vi "Autonomous Independent.vi"() -> ()   [LabVIEW 2017]
doc: "This VI is called when autonomous begins, and will automatically be terminated when autonomous ends. You can carry out timed or sensor driven robot movement independently without needing to return to the caller."
uses:
  <vilib>/Rock Robotics/WPI/ThirdParty/Phoenix-LabVIEW/Motor Controller/Controls/CTRE_Phoenix_MotorControl_ControlMode.ctl
  <vilib>/Rock Robotics/WPI/Utilities/WPI_GetSetVariantRefNum.vi
  <vilib>/Rock Robotics/Network Tables/NT Read String.vi
  <vilib>/Rock Robotics/Network Tables/NT Write Numeric Array.vi
panel:
  in  "Output 6":dbl
  in  "Output 4":dbl
  in  "Output 5":dbl
  in  "Output 3":dbl
  in  "Output 2":dbl
  in  "Ratio":dbl
  in  "Output":dbl
  in  "Ratio 2":dbl
  in  "Acceleration":i32=5000
  in  "Right CV":i32=2000
  in  "PIDF Motion Magic":cluster{"P":dbl, "I":dbl, "D":dbl, "F":dbl}={"P"=0.4, "I"=0.0, "D"=0.0, "F"=0.01}
  in  "Left CV":i32=4000
  # "Be sure to right-click and choose Data Operations>>Make Current Value default if you want to save the array values with the VI"
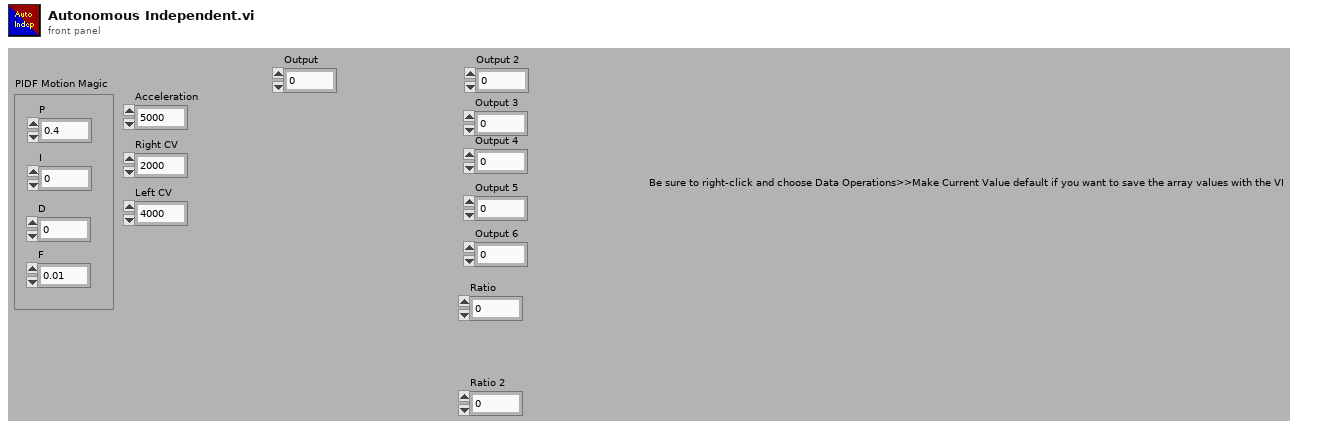
[diagram p1: front panel]
types:
  T1 = typedef "WPI_JoystickDevRef.ctl" = cluster{"Device":T2}
  T2 = typedef "WPI_JoystickDeviceEnum.ctl" = enum16{"USB 0", "USB 1", "USB 2", "USB 3", "USB 4", "USB 5"}
  T3 = typedef "WPI_MotorControlDeviceRef.ctl" = cluster{"DeviceStatus":errorcluster, "Type":T4, "PWM":cluster{"PWM Channel":T5, "DeadBand":T6}, "CAN":cluster{"Device Number":u8, "SetOutput VI Ref":variant, "GetOutput VI Ref":variant, "Enable VI Ref":variant, "Disable VI Ref":variant, "Data":variant}, "Invert":bool, "DIO PWM":cluster{"PWM \"Enable\" Channel":T5, "DIOChannel":T7, "PWM Rate":dbl}}
  T4 = typedef "WPI_MotorControlType.ctl" = enum16{"PWM", "CAN", "DIO PWM"}
  T5 = typedef "FPGA_DIOPWMChannel.ctl" = enum8{"PWM 0", "PWM 1", "PWM 2", "PWM 3", "PWM 4", "PWM 5", "PWM 6", "PWM 7", "PWM 8", "PWM 9", "PWM MXP 0", "PWM MXP 1", "PWM MXP 2", "PWM MXP 3", "PWM MXP 4", "PWM MXP 5", "PWM MXP 6", "PWM MXP 7", "PWM MXP 8", "PWM MXP 9", "Invalid"}
  T6 = typedef "WPI_PWMDeadband.ctl" = cluster{"Name":string, "maxPositivePwm":i32, "minPositivePwm":i32, "centerPwm":i32, "maxNegativePwm":i32, "minNegativePwm":i32, "angularRange":u16}
  T7 = typedef "FPGA_DIOChannel.ctl" = enum8{"DIO 0", "DIO 1", "DIO 2", "DIO 3", "DIO 4", "DIO 5", "DIO 6", "DIO 7", "DIO 8", "DIO 9", "DIO MXP 0", "DIO MXP 1", "DIO MXP 2", "DIO MXP 3", "DIO MXP 4", "DIO MXP 5", "DIO MXP 6", "DIO MXP 7", "DIO MXP 8", "DIO MXP 9", "DIO MXP 10", "DIO MXP 11", "DIO MXP 12", "DIO MXP 13", "DIO MXP 14", "DIO MXP 15", "SPI Port CS1", "SPI Port CS2", "SPI Port CS3", "SPI Port MISO", "SPI Port MOSI", "Invalid"}
  T8 = typedef "CTRE_Phoenix_MotorControl_ControlMode.ctl" = u16
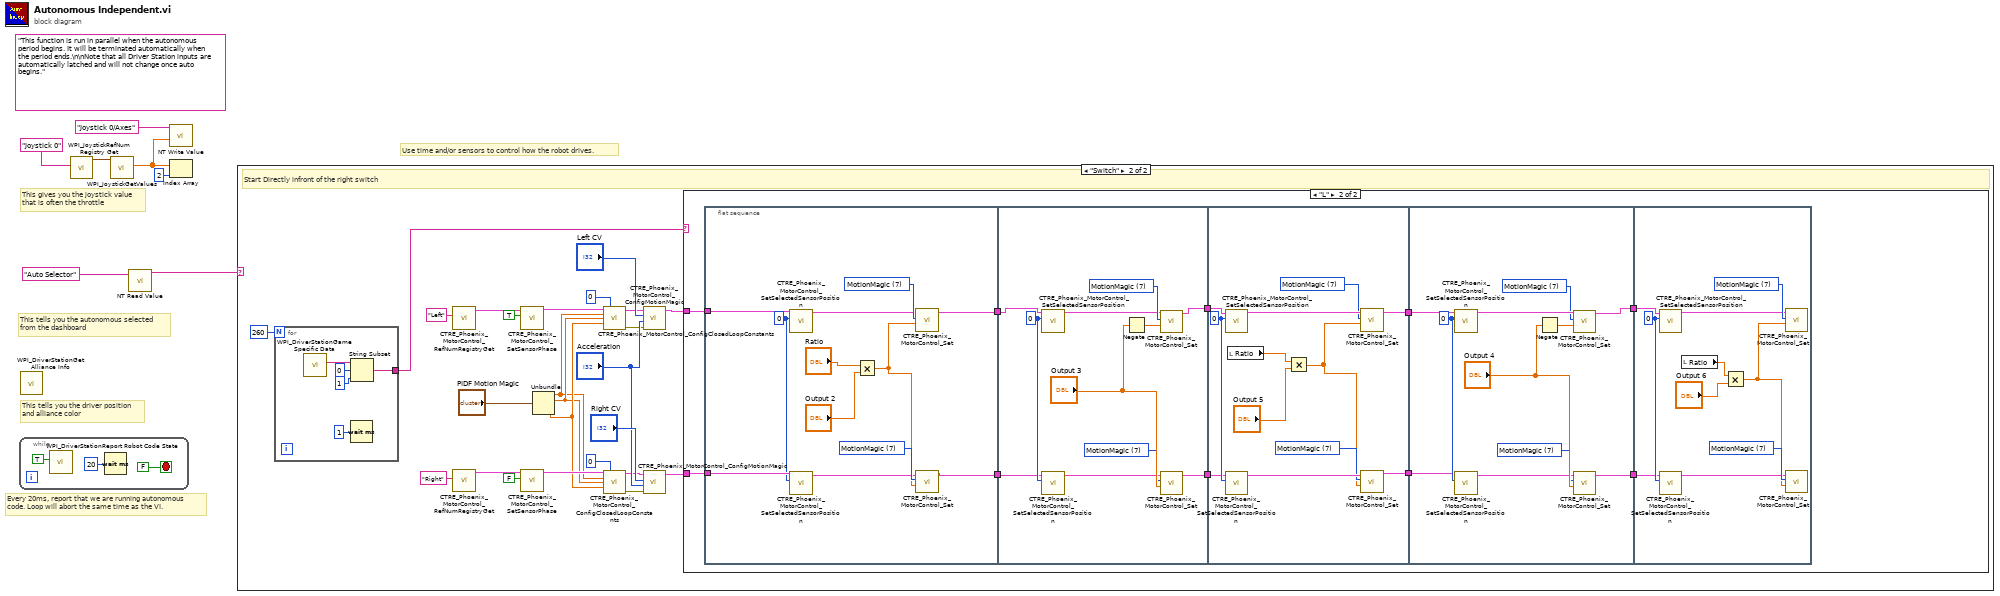
[diagram p0: block diagram]
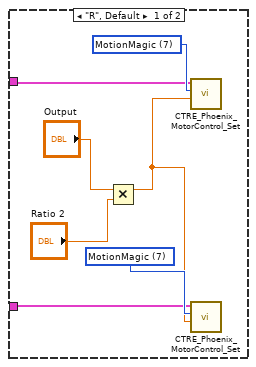
[diagram p3: hidden frame]
diagram:
  (unwired) "This function is run in parallel when the autonomous period begins. It will be terminated automatically when the period ends.\n\nNote that all Driver Station inputs are automatically latched and will not change once auto begins."
  # "This tells you the autonomous selected\nfrom the dashboard"
  # "Every 20ms, report that we are running autonomous\ncode. Loop will abort the same time as the VI."
  # "This gives you the joystick value\nthat is often the throttle"
  # "Use time and/or sensors to control how the robot drives."
  # "This tells you the driver position\nand alliance color"
  n1 = while {
    stop <- FALSE stop-if-true
    n2 = call <vilib>:"WPI_DriverStationReport Robot Code State.vi"("Autonomous"=TRUE) -> ()  [unwired: 10 in, 1 out]
    n3 = Wait (ms)(milliseconds to wait=u32 20) -> ()  [unwired: 1 out]
  }
  n4 = call <vilib>:"WPI_DriverStationGet Alliance Info.vi"() -> ()  [unwired: 12 out]
  n5 = call <vilib>:"WPI_JoystickRefNum Registry Get.vi"("refnum name"="Joystick 0") -> ("JoystickDevRef"=w6:T1)  [unwired: 1 in, 9 out]
  n6 = call <vilib>:"WPI_JoystickGetValues.vi"("JoystickDevRef"=w6) -> ("Axes"=w3:dbl[])  [unwired: 6 in, 4 out]
  n7 = call-poly <vilib>:"NT Read Value.vi"("Name"="Auto Selector") -> ("String"=w1:string)  [unwired: 9 in, 1 out]
  n8 = call-poly <vilib>:"NT Write Value.vi"("Numeric Array"=w3, "Name"="Joystick 0/Axes") -> ()  [unwired: 9 in, 1 out]
  n9 = Index Array(array=w3, index=2) -> ()  [unwired: 1 out]
  n10 = case shown="\"Switch\"" w1 {
    frame Default {
      # "You can put your main auto here, or you can right-click on the case and make any\nother frame be the default case."
      # "This is the frame that will execute if no selection is made, or if it is not recognized"
    }
    frame "Switch" {
      # "Start Directly infront of the right switch"
      n11 = for {
        N: 260 -> [_]
        tunnel: [w37] -> w35
        n12 = call <vilib>:"WPI_DriverStationGame Specific Data.vi"() -> ("Game Specific Data"=w40:string)  [unwired: 11 in]
        n13 = Wait (ms)(milliseconds to wait=u32 1) -> ()  [unwired: 1 out]
        n14 = String Subset(string=w40, offset (0)=0, length (rest)=1 ("length (rest)")) -> (substring=w37:string)
      }
      n15 = call "CTRE_Phoenix_MotorControl_RefNumRegistryGet.vi"("refnum name"="Left") -> ("PhoenixMotorControlDevRef"=w19:T3)  [unwired: 9 in, 1 out]
      n16 = call "CTRE_Phoenix_MotorControl_RefNumRegistryGet.vi"("refnum name"="Right") -> ("PhoenixMotorControlDevRef"=w20:T3)  [unwired: 9 in, 1 out]
      n17 = call "CTRE_Phoenix_MotorControl_SetSensorPhase.vi"("PhaseSensor"=TRUE, "PhoenixMotorControlDevRef"=w19) -> ("PhoenixMotorControlDevRef"=w33:T3)  [unwired: 8 in, 1 out]
      n18 = call "CTRE_Phoenix_MotorControl_SetSensorPhase.vi"("PhaseSensor"=FALSE, "PhoenixMotorControlDevRef"=w20) -> ("PhoenixMotorControlDevRef"=w32:T3)  [unwired: 8 in, 1 out]
      n19 = Unbundle("PIDF Motion Magic") -> ("P"=w25:dbl, "I"=w26:dbl, "D"=w27:dbl)  [unwired: 1 out]
      n20 = call "CTRE_Phoenix_MotorControl_ConfigClosedLoopConstants.vi"("PhoenixMotorControlDevRef"=w33, "slotIdx"=0, "P"=w25, "I"=w26, "D"=w27) -> ("PhoenixMotorControlDevRef"=w21:T3, "error out"=w22:errorcluster)  [unwired: 9 in]
      n21 = call "CTRE_Phoenix_MotorControl_ConfigClosedLoopConstants.vi"("PhoenixMotorControlDevRef"=w32, "slotIdx"=0, "P"=w25, "I"=w26, "D"=w27) -> ("PhoenixMotorControlDevRef"=w23:T3, "error out"=w24:errorcluster)  [unwired: 9 in]
      n22 = call "CTRE_Phoenix_MotorControl_ConfigMotionMagic.vi"("error in (no error)"=w22, "Acceleration"="Acceleration", "Cruise Velocity"="Left CV", "PhoenixMotorControlDevRef"=w21) -> ("PhoenixMotorControlDevRef"=w11:T3)  [unwired: 6 in, 1 out]
      n23 = call "CTRE_Phoenix_MotorControl_ConfigMotionMagic.vi"("error in (no error)"=w24, "Acceleration"="Acceleration", "Cruise Velocity"="Right CV", "PhoenixMotorControlDevRef"=w23) -> ("PhoenixMotorControlDevRef"=w12:T3)  [unwired: 6 in, 1 out]
      n24 = case shown="\"L\"" w35 {
        tunnel: w12 -> [w44 w57]
        tunnel: w11 -> [w43 w56]
        frame "R", Default {
          w46 = T8 7 items=["PercentOutput"=0, "Position"=1, "Velocity"=2, "Current"=3, "Follower"=5, "MotionProfile"=6, "MotionMagic"=7, "MotionMagicArc"=8, "MotionProfileArc"=10, "Disabled"=15] ("Control Mode")
          w45 = T8 7 items=["PercentOutput"=0, "Position"=1, "Velocity"=2, "Current"=3, "Follower"=5, "MotionProfile"=6, "MotionMagic"=7, "MotionMagicArc"=8, "MotionProfileArc"=10, "Disabled"=15] ("Control Mode")
          n25 = Multiply(x="Output", y="Ratio 2") -> (x*y=w42:dbl)
          n26 = call "CTRE_Phoenix_MotorControl_Set.vi"("Output"=w42, "Control Mode"=w45, "PhoenixMotorControlDevRef"=w43) -> ()  [unwired: 7 in, 2 out]
          n27 = call "CTRE_Phoenix_MotorControl_Set.vi"("Output"=w42, "Control Mode"=w46, "PhoenixMotorControlDevRef"=w44) -> ()  [unwired: 7 in, 2 out]
        }
        frame "L" {
          n28 = flat-sequence {
            tunnel: w57 -> [w63]
            tunnel: w56 -> [w65]
            tunnel: [w67] -> w55
            tunnel: [w66] -> w54
            tunnel: w55 -> [w72]
            tunnel: w54 -> [w75]
            tunnel: [w71] -> w51
            tunnel: [w70] -> w50
            tunnel: [w87] -> w53
            tunnel: [w86] -> w52
            tunnel: w51 -> [w85]
            tunnel: w50 -> [w84]
            tunnel: w53 -> [w96]
            tunnel: w52 -> [w95]
            tunnel: [w94] -> w49
            tunnel: [w93] -> w48
            tunnel: w49 -> [w108]
            tunnel: w48 -> [w107]
            frame #0 {
              w61 = 0 ("New Sensor Position")
              w69 = T8 7 items=["PercentOutput"=0, "Position"=1, "Velocity"=2, "Current"=3, "Follower"=5, "MotionProfile"=6, "MotionMagic"=7, "MotionMagicArc"=8, "MotionProfileArc"=10, "Disabled"=15] ("Control Mode")
              w68 = T8 7 items=["PercentOutput"=0, "Position"=1, "Velocity"=2, "Current"=3, "Follower"=5, "MotionProfile"=6, "MotionMagic"=7, "MotionMagicArc"=8, "MotionProfileArc"=10, "Disabled"=15] ("Control Mode")
              n29 = call "CTRE_Phoenix_MotorControl_SetSelectedSensorPosition.vi"("New Sensor Position"=w61, "PhoenixMotorControlDevRef"=w65) -> ("PhoenixMotorControlDevRef"=w64:T3)  [unwired: 8 in, 1 out]
              n30 = call "CTRE_Phoenix_MotorControl_SetSelectedSensorPosition.vi"("New Sensor Position"=w61, "PhoenixMotorControlDevRef"=w63) -> ("PhoenixMotorControlDevRef"=w62:T3)  [unwired: 8 in, 1 out]
              n31 = Multiply(x="Ratio", y="Output 2") -> (x*y=w59:dbl)
              n32 = call "CTRE_Phoenix_MotorControl_Set.vi"("Output"=w59, "Control Mode"=w68, "PhoenixMotorControlDevRef"=w64) -> ("PhoenixMotorControlDevRef"=w66:T3)  [unwired: 7 in, 1 out]
              n33 = call "CTRE_Phoenix_MotorControl_Set.vi"("Output"=w59, "Control Mode"=w69, "PhoenixMotorControlDevRef"=w62) -> ("PhoenixMotorControlDevRef"=w67:T3)  [unwired: 7 in, 1 out]
            }
            frame #1 {
              w76 = 0 ("New Sensor Position")
              w79 = T8 7 items=["PercentOutput"=0, "Position"=1, "Velocity"=2, "Current"=3, "Follower"=5, "MotionProfile"=6, "MotionMagic"=7, "MotionMagicArc"=8, "MotionProfileArc"=10, "Disabled"=15] ("Control Mode")
              w78 = T8 7 items=["PercentOutput"=0, "Position"=1, "Velocity"=2, "Current"=3, "Follower"=5, "MotionProfile"=6, "MotionMagic"=7, "MotionMagicArc"=8, "MotionProfileArc"=10, "Disabled"=15] ("Control Mode")
              n34 = call "CTRE_Phoenix_MotorControl_SetSelectedSensorPosition.vi"("New Sensor Position"=w76, "PhoenixMotorControlDevRef"=w75) -> ("PhoenixMotorControlDevRef"=w74:T3)  [unwired: 8 in, 1 out]
              n35 = call "CTRE_Phoenix_MotorControl_SetSelectedSensorPosition.vi"("New Sensor Position"=w76, "PhoenixMotorControlDevRef"=w72) -> ("PhoenixMotorControlDevRef"=w73:T3)  [unwired: 8 in, 1 out]
              n36 = Negate(x="Output 3") -> (-x=w77:dbl)
              n37 = call "CTRE_Phoenix_MotorControl_Set.vi"("Output"=w77, "Control Mode"=w78, "PhoenixMotorControlDevRef"=w74) -> ("PhoenixMotorControlDevRef"=w70:T3)  [unwired: 7 in, 1 out]
              n38 = call "CTRE_Phoenix_MotorControl_Set.vi"("Output"="Output 3", "Control Mode"=w79, "PhoenixMotorControlDevRef"=w73) -> ("PhoenixMotorControlDevRef"=w71:T3)  [unwired: 7 in, 1 out]
            }
            frame #2 {
              w92 = 0 ("New Sensor Position")
              w88 = T8 7 items=["PercentOutput"=0, "Position"=1, "Velocity"=2, "Current"=3, "Follower"=5, "MotionProfile"=6, "MotionMagic"=7, "MotionMagicArc"=8, "MotionProfileArc"=10, "Disabled"=15] ("Control Mode")
              w89 = T8 7 items=["PercentOutput"=0, "Position"=1, "Velocity"=2, "Current"=3, "Follower"=5, "MotionProfile"=6, "MotionMagic"=7, "MotionMagicArc"=8, "MotionProfileArc"=10, "Disabled"=15] ("Control Mode")
              n39 = call "CTRE_Phoenix_MotorControl_SetSelectedSensorPosition.vi"("New Sensor Position"=w92, "PhoenixMotorControlDevRef"=w84) -> ("PhoenixMotorControlDevRef"=w90:T3)  [unwired: 8 in, 1 out]
              n40 = call "CTRE_Phoenix_MotorControl_SetSelectedSensorPosition.vi"("New Sensor Position"=w92, "PhoenixMotorControlDevRef"=w85) -> ("PhoenixMotorControlDevRef"=w91:T3)  [unwired: 8 in, 1 out]
              n41 = local read "Ratio"() -> (w81:dbl)
              n42 = Multiply(x=w81, y="Output 5") -> (x*y=w82:dbl)
              n43 = call "CTRE_Phoenix_MotorControl_Set.vi"("Output"=w82, "Control Mode"=w89, "PhoenixMotorControlDevRef"=w90) -> ("PhoenixMotorControlDevRef"=w87:T3)  [unwired: 7 in, 1 out]
              n44 = call "CTRE_Phoenix_MotorControl_Set.vi"("Output"=w82, "Control Mode"=w88, "PhoenixMotorControlDevRef"=w91) -> ("PhoenixMotorControlDevRef"=w86:T3)  [unwired: 7 in, 1 out]
            }
            frame #3 {
              w99 = 0 ("New Sensor Position")
              w98 = T8 7 items=["PercentOutput"=0, "Position"=1, "Velocity"=2, "Current"=3, "Follower"=5, "MotionProfile"=6, "MotionMagic"=7, "MotionMagicArc"=8, "MotionProfileArc"=10, "Disabled"=15] ("Control Mode")
              w97 = T8 7 items=["PercentOutput"=0, "Position"=1, "Velocity"=2, "Current"=3, "Follower"=5, "MotionProfile"=6, "MotionMagic"=7, "MotionMagicArc"=8, "MotionProfileArc"=10, "Disabled"=15] ("Control Mode")
              n45 = call "CTRE_Phoenix_MotorControl_SetSelectedSensorPosition.vi"("New Sensor Position"=w99, "PhoenixMotorControlDevRef"=w96) -> ("PhoenixMotorControlDevRef"=w101:T3)  [unwired: 8 in, 1 out]
              n46 = call "CTRE_Phoenix_MotorControl_SetSelectedSensorPosition.vi"("New Sensor Position"=w99, "PhoenixMotorControlDevRef"=w95) -> ("PhoenixMotorControlDevRef"=w100:T3)  [unwired: 8 in, 1 out]
              n47 = Negate(x="Output 4") -> (-x=w102:dbl)
              n48 = call "CTRE_Phoenix_MotorControl_Set.vi"("Output"=w102, "Control Mode"=w97, "PhoenixMotorControlDevRef"=w101) -> ("PhoenixMotorControlDevRef"=w94:T3)  [unwired: 7 in, 1 out]
              n49 = call "CTRE_Phoenix_MotorControl_Set.vi"("Output"="Output 4", "Control Mode"=w98, "PhoenixMotorControlDevRef"=w100) -> ("PhoenixMotorControlDevRef"=w93:T3)  [unwired: 7 in, 1 out]
            }
            frame #4 {
              w109 = 0 ("New Sensor Position")
              w113 = T8 7 items=["PercentOutput"=0, "Position"=1, "Velocity"=2, "Current"=3, "Follower"=5, "MotionProfile"=6, "MotionMagic"=7, "MotionMagicArc"=8, "MotionProfileArc"=10, "Disabled"=15] ("Control Mode")
              w112 = T8 7 items=["PercentOutput"=0, "Position"=1, "Velocity"=2, "Current"=3, "Follower"=5, "MotionProfile"=6, "MotionMagic"=7, "MotionMagicArc"=8, "MotionProfileArc"=10, "Disabled"=15] ("Control Mode")
              n50 = call "CTRE_Phoenix_MotorControl_SetSelectedSensorPosition.vi"("New Sensor Position"=w109, "PhoenixMotorControlDevRef"=w108) -> ("PhoenixMotorControlDevRef"=w111:T3)  [unwired: 8 in, 1 out]
              n51 = call "CTRE_Phoenix_MotorControl_SetSelectedSensorPosition.vi"("New Sensor Position"=w109, "PhoenixMotorControlDevRef"=w107) -> ("PhoenixMotorControlDevRef"=w110:T3)  [unwired: 8 in, 1 out]
              n52 = local read "Ratio"() -> (w105:dbl)
              n53 = Multiply(x=w105, y="Output 6") -> (x*y=w104:dbl)
              n54 = call "CTRE_Phoenix_MotorControl_Set.vi"("Output"=w104, "Control Mode"=w112, "PhoenixMotorControlDevRef"=w111) -> ()  [unwired: 7 in, 2 out]
              n55 = call "CTRE_Phoenix_MotorControl_Set.vi"("Output"=w104, "Control Mode"=w113, "PhoenixMotorControlDevRef"=w110) -> ()  [unwired: 7 in, 2 out]
            }
          }
        }
      }
    }
  }
